vi "ProjectUndeploy.vi"(8 "error in (no error)":errorcluster) -> (0 "error out":errorcluster)   [LabVIEW 2015, in "MiscHelperVIs.lvlib"]
uses:
  MiscHelperVIs.lvlib
  <vilib>/NI Veristand/Execution/Project/NI_VS Project ExecutionAPI.lvlib
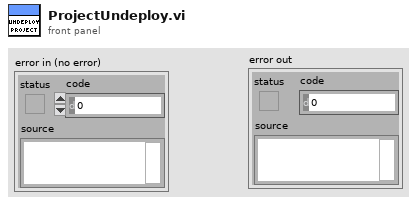
[diagram p1: front panel]
types:
  T1 = typedef "MiscHelperVIs.lvlib/VeriStand dotNet References.ctl" = cluster{"VS Project .NET Refnum":refnum<k24>, "Workspace Manager .NET Refnum":refnum<k24>}
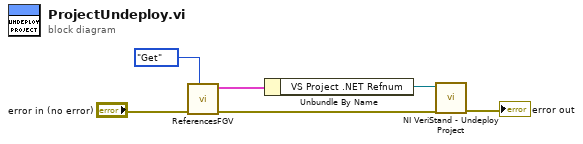
[diagram p0: block diagram]
diagram:
  n1 = call "ReferencesFGV.vi"("Get/Set"=enum16{"Get", "Set"}."Get", "error in (no error)"="error in (no error)") -> ("error out"=w1:errorcluster, "VeriStand dotNET Refs out"=w4:T1)  [unwired: 8 in]
  n2 = Unbundle By Name(w4) -> ("VS Project .NET Refnum"=w2:refnum<k24>)
  n3 = call <vilib>:"NI VeriStand - Undeploy Project.vi"("error in (no error)"=w1, "Project Ref in"=w2) -> ("error out"=→"error out":errorcluster)  [unwired: 8 in, 1 out]
